vi "SLL DE View Datalog File.vi"(8 "error in(no error)":errorcluster) -> (0 "error Out":errorcluster)   [LabVIEW 2013]
uses:
  Controls/SLL DE Virtual Graph Options.ctl
  Controls/SLL DE Get Plot LV2Global Options.ctl
  Controls/SLL DE Virtual Chart Datalog Driver Options.ctl
  <vilib>/Utility/miscctls.llb/LVAnnotationListTypeDef.ctl
  Controls/SLL DE Get Plot LV2Global Parameters.ctl
panel:
  out "Time :":string="02:30:20 PM"
  out "Date :":string="08-30-2009"
  in  "Import":bool caption="Exit"
  in  "Plot 4":u16(ring) caption="Y-Axis(1)" items=["None"]
  in  "Plot 3":u16(ring) caption="Y-Axis(1)" items=["None"]
  in  "Plot 2":u16(ring) caption="Y-Axis(1)" items=["None"]
  in  "Y-Axis 2":bool=TRUE
  in  "Y-Axis 1":bool=TRUE
  in  "Plot 1":u16(ring) caption="Y-Axis(1)" items=["None"]
  in  "X-Scale":u16(ring) caption="Y-Axis(1)"
  out "Graph":T1(graph)
  in  "Importing File Path":path=path "D:/STI Projects/DAQ Engine/SLL DAQ Engine/Software/Info/Report/Log_08_2009_30_13_15_39.csv"
  in  "Data Cluster":T3={"Record"=FALSE, "Datalog Folder Path"=path "D:/Projects/Projects/Eaton Prop Valve Test Stand/Software/Info/Datalog File Path/Back up.dat", "Graph - Interval b/w Samples"=0, "AI Sampling Rate (Samples/Sec)"=3.0, "Data Log To csv File"=[], "File - Interval b/w Samples"=0, "Time Array"=[], "Graph Mod"=0, "File Mod"=0, "Plot Details"={"Sample Value In"=[], "Plot 1"=FALSE, "Plot 2"=FALSE, "Plot 3"=FALSE, "Plot 4"=FALSE}, "Channel Names"=[]}
  in  "Snap Shot":bool caption="Duplicate SupFile"
  in  "Exit":bool
  in  "Print":bool
  # "Logo"
  # "<Project Name>"
  # "Datalog File Display"
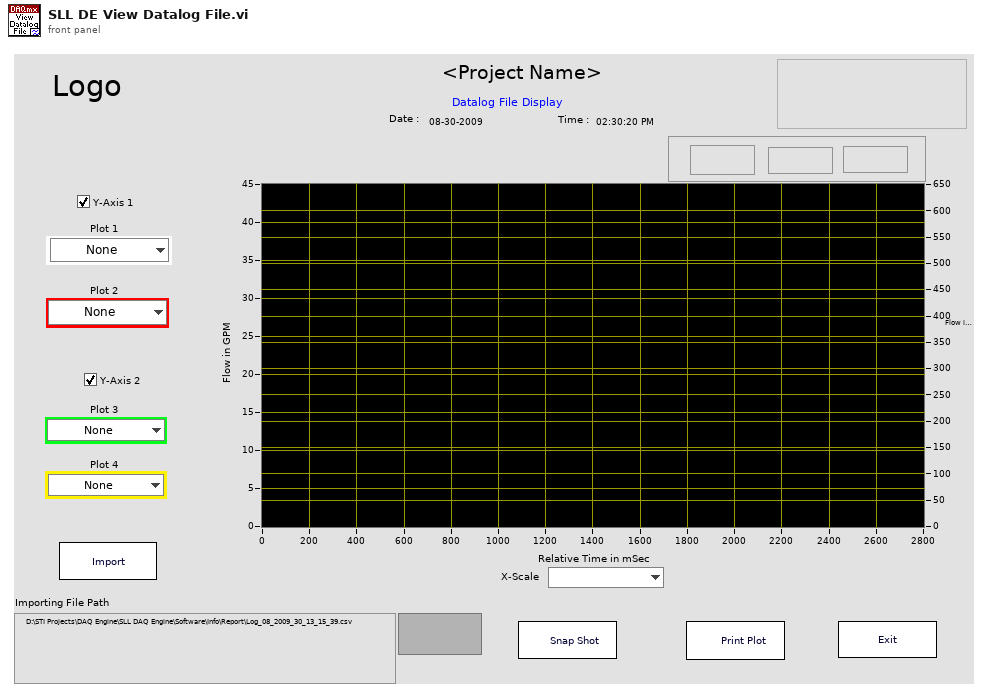
[diagram p1: front panel]
types:
  T1 = cluster{"Sample Value In":sgl[], "Sample Value In":sgl[]}[]
  T2 = typedef "SLL DE Get Plot LV2Global Parameters.ctl" = cluster{"Sample Value In":sgl[][], "Plot 1":bool, "Plot 2":bool, "Plot 3":bool, "Plot 4":bool}
  T3 = cluster{"Record":bool, "Datalog Folder Path":path, "Graph - Interval b/w Samples":i32, "AI Sampling Rate (Samples/Sec)":dbl, "Data Log To csv File":dbl[][], "File - Interval b/w Samples":i32, "Time Array":timestamp[], "Graph Mod":i32, "File Mod":i32, "Plot Details":T2, "Channel Names":string[]}
  T4 = typedef "SLL DE Virtual Graph Options.ctl" = enum16{"Initialize", "Initialize Channel List", "Check Channel Type", "Update Graph Parameters", "Poll Events", "Get Values", "Config Plot", "Plot Ramp", "Datalog", "Add Plot Name", "Enable Record", "Snap Shot", "Restart", "Print Plot", "Error", "Exit"}
  T5 = typedef "SLL DE Get Plot LV2Global Options.ctl" = enum16{"Init", "Get Plot", "Read Plot"}
  T6 = typedef "SLL DE Virtual Chart Datalog Driver Options.ctl" = enum16{"Initialise", "Write Headings", "Write", "Check File Size", "Read", "Clear"}
  T7 = cluster{"Name":string, "Color":u32, "Style":u8, "Point Style":u8, "Name Visible":bool, "Allow Drag":bool, "Annotation Mode":u32, "Plot":i32, "Index":i32, "Position":cluster{"X":dbl, "Y":dbl}, "X Scale":u32, "Y Scale":u32, "Show Arrow":bool, "Lock Name":bool, "Plot Area":i32, "Label Offset":cluster{"X":dbl, "Y":dbl}}[]
  T8 = cluster{"Name":string, "Color":u32, "Style":u8, "Point Style":u8, "Name Visible":bool, "Allow Drag":bool, "Annotation Mode":u32, "Plot":i32, "Index":i32, "Position":cluster{"X":dbl, "Y":dbl}, "X Scale":u32, "Y Scale":u32, "Show Arrow":bool, "Lock Name":bool, "Plot Area":i32, "Label Offset":cluster{"X":dbl, "Y":dbl}}
  T9 = cluster{"Plot 1":string, "Plot 2":string, "Plot 3":string, "Plot 4":string, "X Scale":string, "Y-Axis 2":bool, "Y-Axis 1":bool}
  T10 = typedef "LVAnnotationListTypeDef.ctl" = cluster{"Name":string, "Color":u32, "Style":u8, "Point Style":u8, "Name Visible":bool, "Allow Drag":bool, "Annotation Mode":u32, "Plot":i32, "Index":i32, "Position":cluster{"X":dbl, "Y":dbl}, "X Scale":u32, "Y Scale":u32, "Show Arrow":bool, "Lock Name":bool, "Plot Area":i32, "Label Offset":cluster{"X":dbl, "Y":dbl}}[]
  T11 = typedef "SLL DE List of AI Channel Type.ctl" = enum16{"Pressure", "Flow", "Temperature", "Time Scale", "Voltage", "Current", "Frequency", "Sound", "Speed", "Torque", "Distance", "Channel Type 1", "Channel Type 2", "Channel Type 3"}
  T12 = cluster{"Time Scale":sgl[], "Sample Value In":sgl[]}[]
  T13 = enum16{"Left Button", "Center Button", "Right Button", "Window Close"}
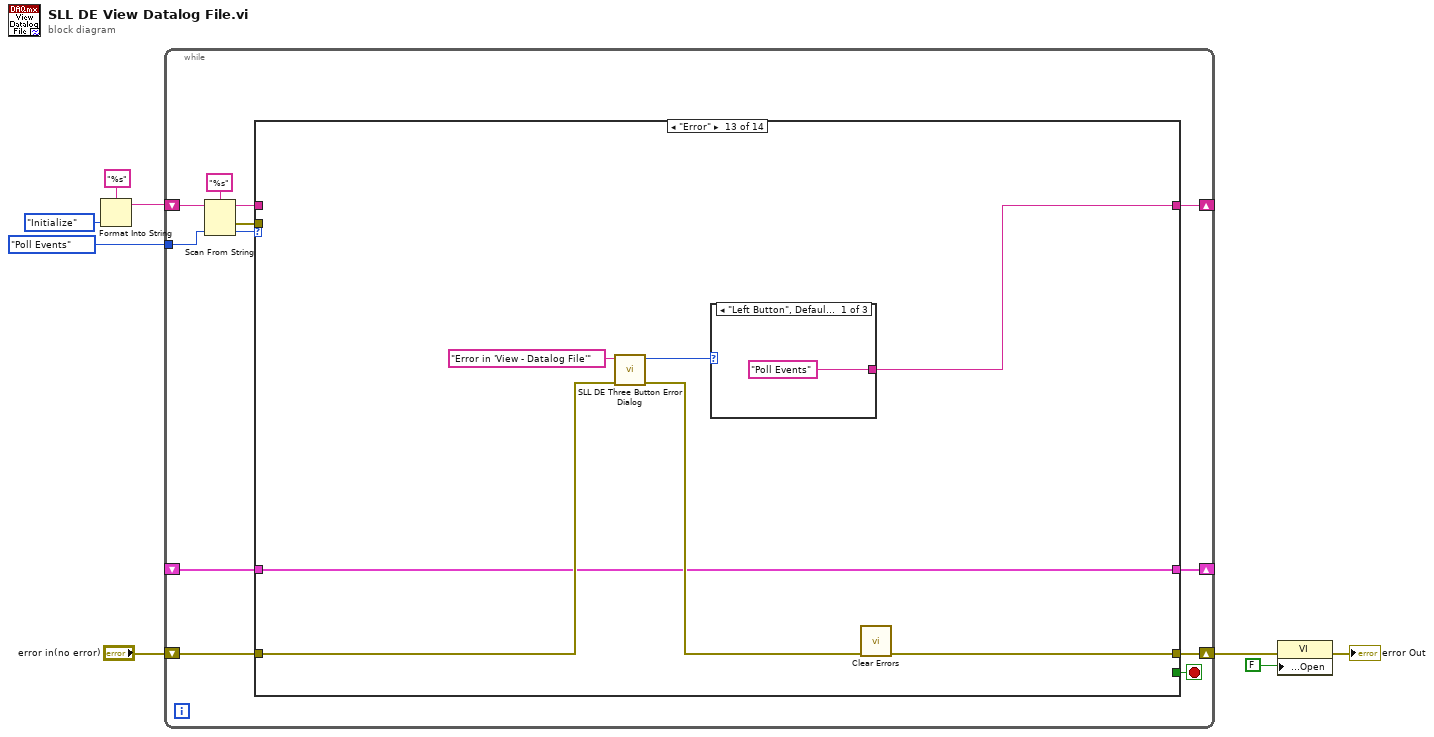
[diagram p0: block diagram]
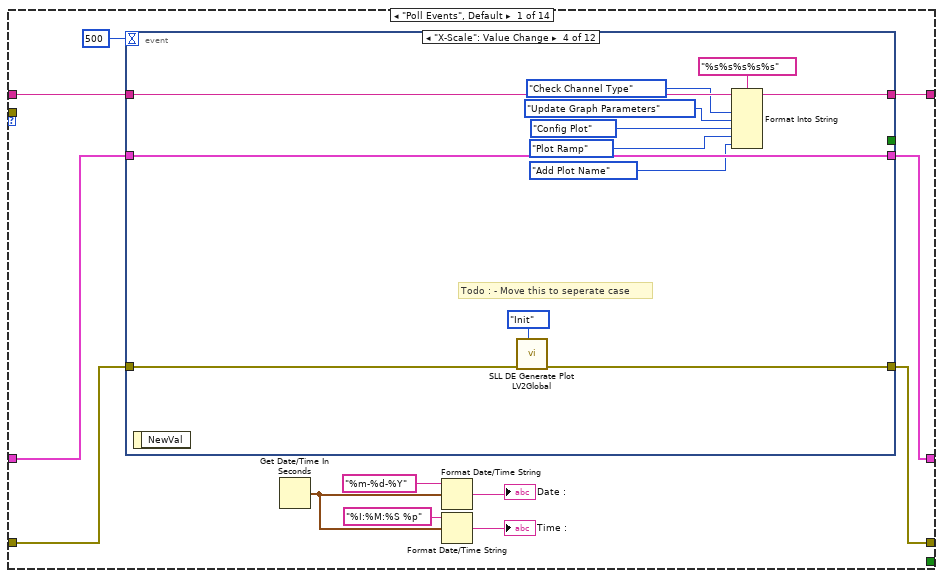
[diagram p2: hidden frame]
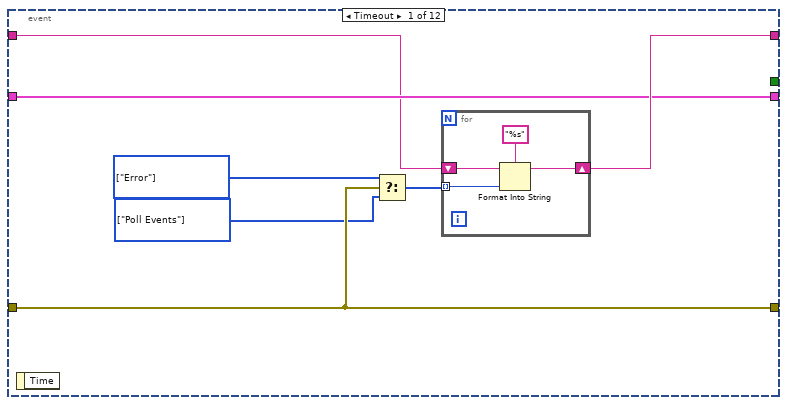
[diagram p3: hidden frame]
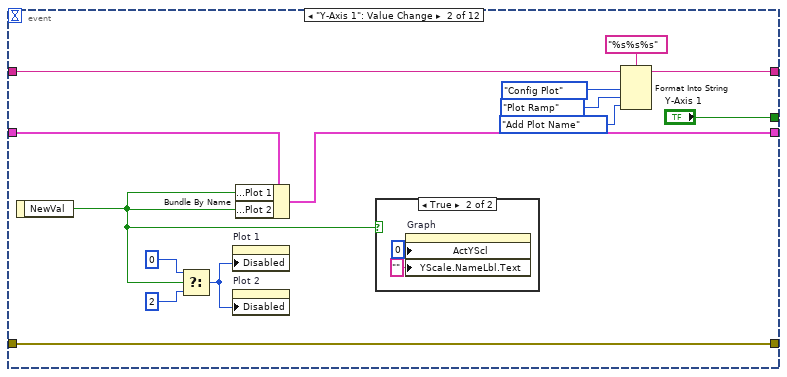
[diagram p4: hidden frame]
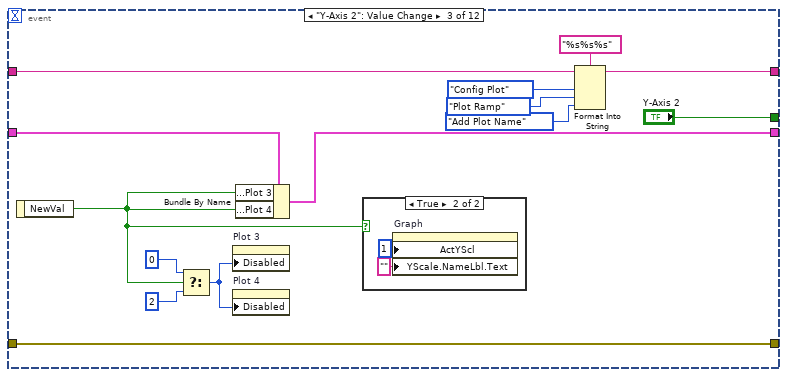
[diagram p6: hidden frame]
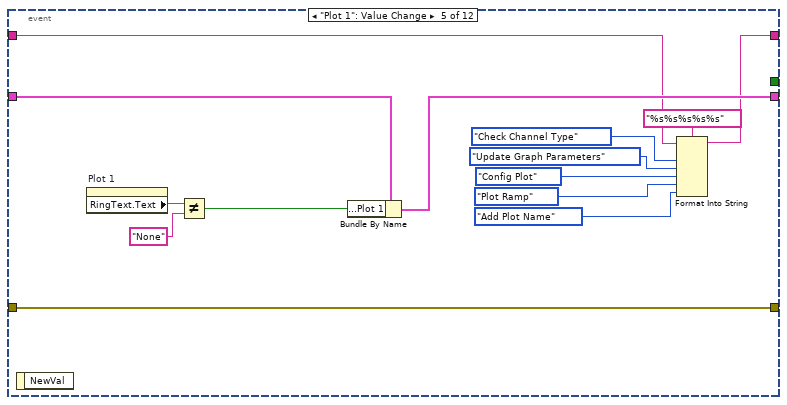
[diagram p8: hidden frame]
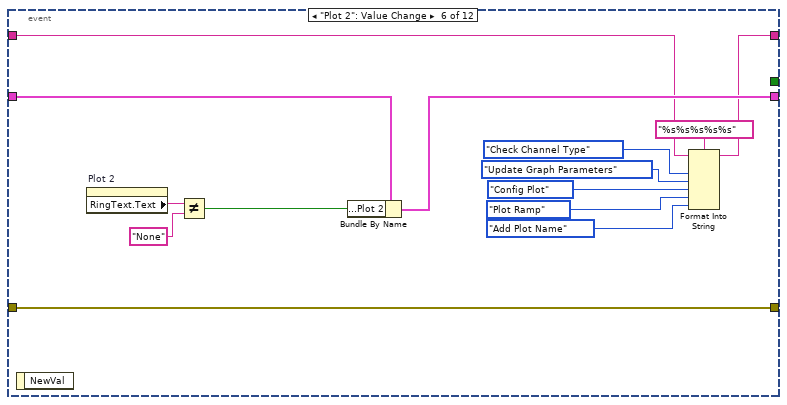
[diagram p9: hidden frame]
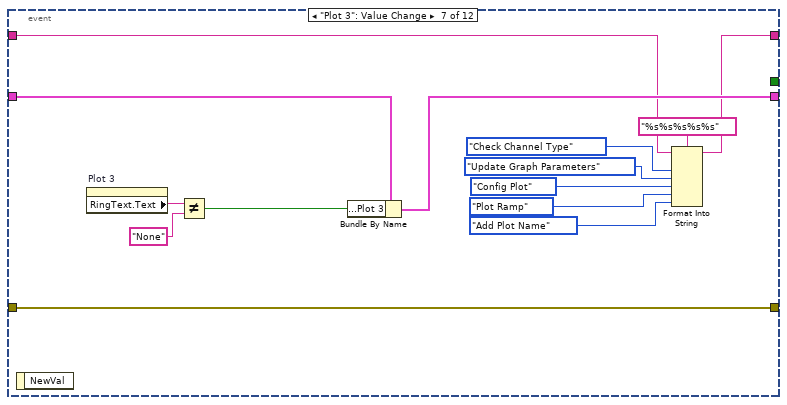
[diagram p10: hidden frame]
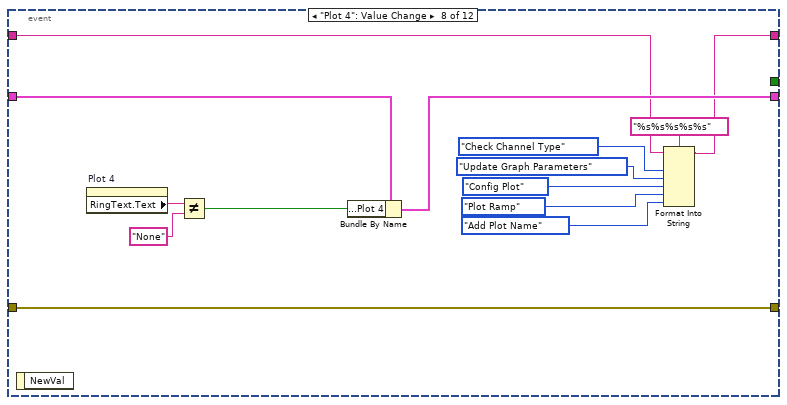
[diagram p11: hidden frame]
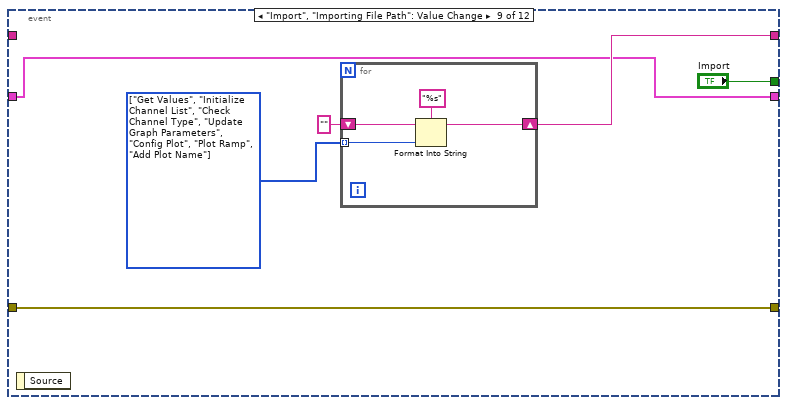
[diagram p12: hidden frame]
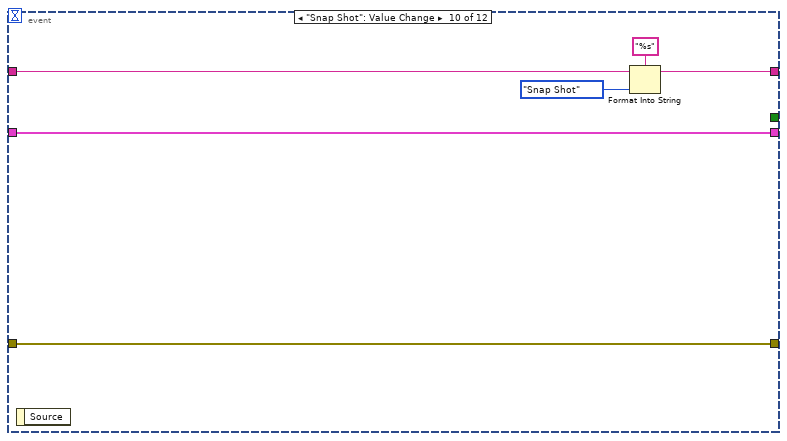
[diagram p13: hidden frame]
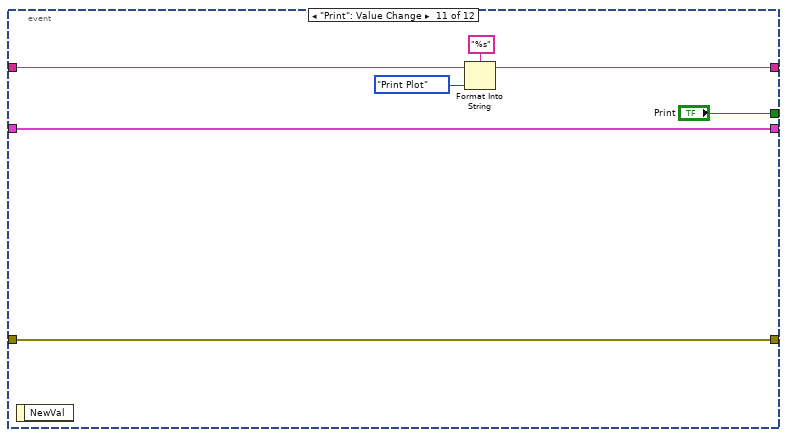
[diagram p14: hidden frame]
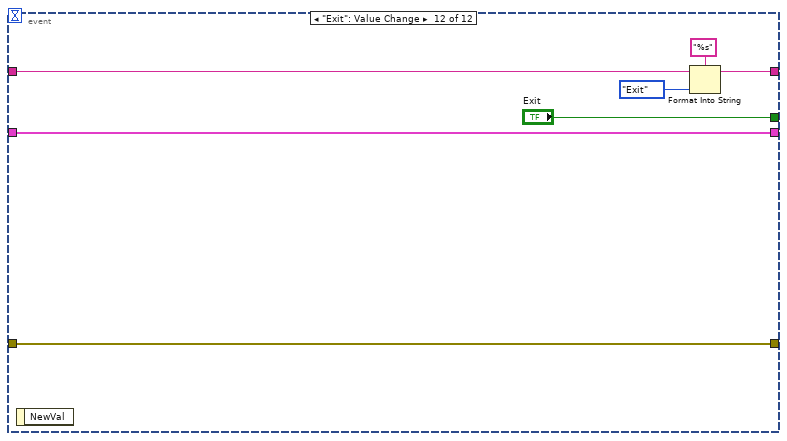
[diagram p15: hidden frame]
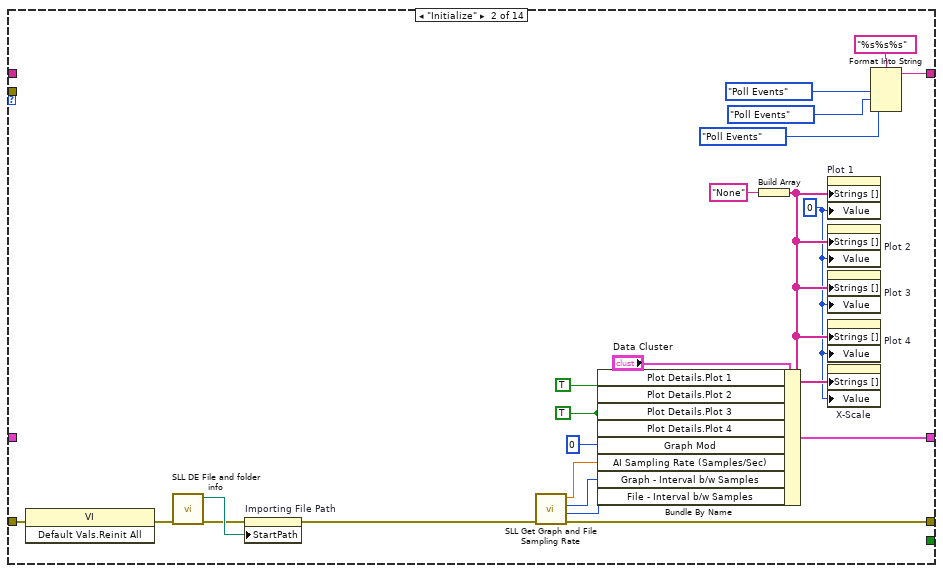
[diagram p16: hidden frame]
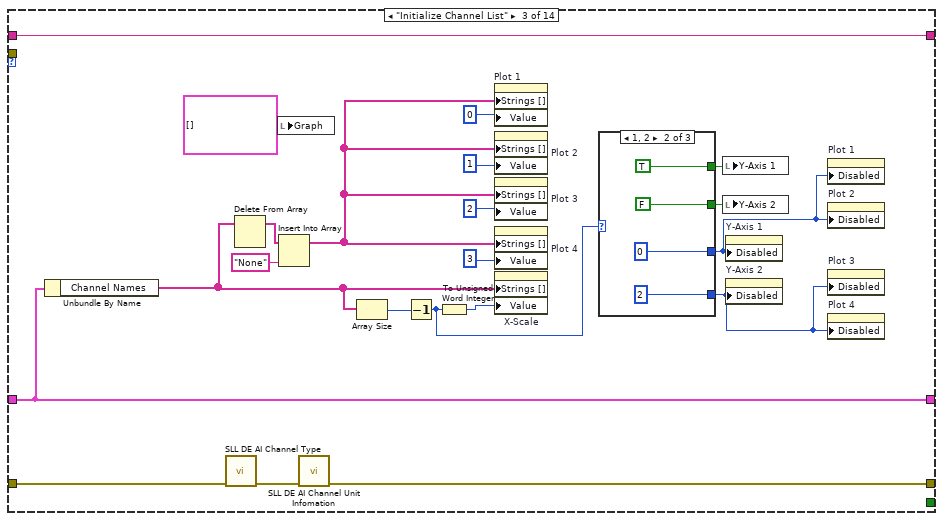
[diagram p17: hidden frame]
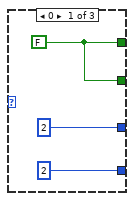
[diagram p18: hidden frame]
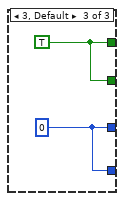
[diagram p19: hidden frame]
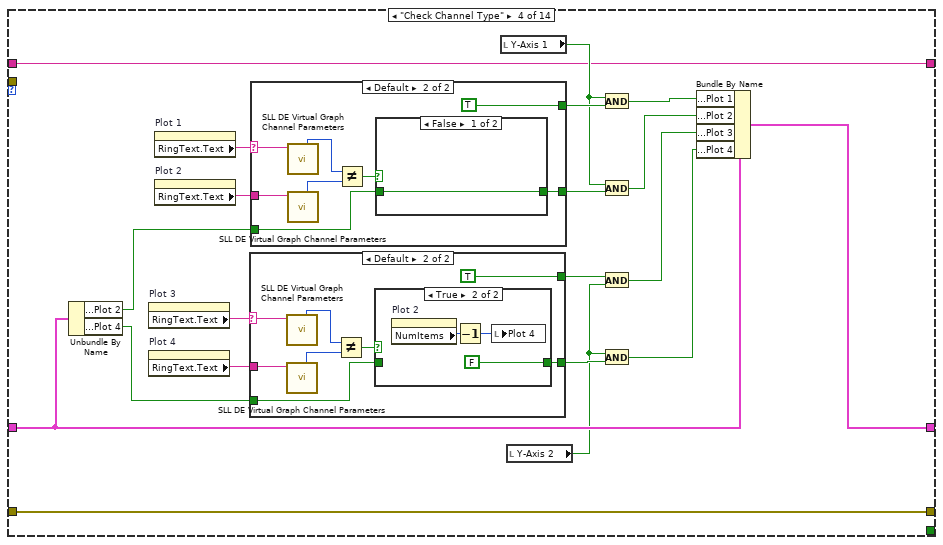
[diagram p20: hidden frame]
diagram:
  n1 = Format Into String(format string="%s", SLL_DE_Virtual_Graph_Options."Initialize" ("SLL DE Virtual Chart Options")) -> (resulting string=w8:string)  [unwired: 2 in, 1 out]
  n2 = while {
    shift-right: [w17] -> _
    shift-left: w8 -> [w20]
    shift-right: [w16] -> _
    shift-left: _ -> [w14]
    shift-right: [w13] -> w6
    shift-left: "error in(no error)" -> [w12]
    tunnel: SLL_DE_Virtual_Graph_Options."Poll Events" ("SLL DE Virtual Chart Options") -> [w10]
    stop <- w15 stop-if-true
    n3 = Scan From String(format string="%s", input string=w20, default 1=w10) -> (remaining string=w18:string, error out=w11:errorcluster, output 1=w19:T4)  [unwired: 2 in, 1 out]
    n4 = case shown="\"Error\"" w19 {
      tunnel: w18 -> [w31 _ w208 w226 w274 w313 w320 w334 w353 w388 w403 w419 _ w437]
      tunnel: [w30 w188 w208 w226 w274 w313 w320 w334 w353 w388 w403 w419 w421 w437] -> w17
      tunnel: [w28 w192 w198 w237 w278 w314 w319 w331 w336 w387 w391 w408 w422 w436] -> w16
      tunnel: [_ _ _ _ _ _ _ _ _ FALSE _ _ _ TRUE] -> w15
      tunnel: w14 -> [w29 _ w198 w238 w278 w312 w319 w331 w336 w387 w391 w408 w422 w436]
      tunnel: [w26 w180 w201 w245 w277 w308 w324 w332 w337 w383 w390 w404 w420 w432] -> w13
      tunnel: w12 -> [w27 w195 w203 w245 w279 w311 w317 w333 w338 w384 w392 w409 w424 w433]
      tunnel: w11 -> [_ _ _ _ _ _ _ _ _ _ _ _ _ _]
      frame "Poll Events", Default {
        n5 = event shown="[3] \"X-Scale\": Value Change" {
          selector: _ -> [_ _ _ _ _ _ _ _ _ _ _ _]
          dyn-events: _ -> [_ _ _ _ _ _ _ _ _ _ _ _]
          timeout: 500 -> [_ _ _ _ _ _ _ _ _ _ _ _]
          tunnel: w31 -> [w34 w52 w62 w80 w90 w104 w117 w130 _ w156 w160 w167]
          tunnel: [w39 w53 w61 w79 w89 w103 w116 w131 w145 w157 w164 w172] -> w30
          tunnel: [_ "Y-Axis 1" "Y-Axis 2" _ _ _ _ _ "Import" _ "Print" "Exit"] -> _
          tunnel: w29 -> [w38 w56 w67 w84 w101 w112 w126 w140 w144 w155 w163 w170]
          tunnel: [w38 w55 w68 w84 w100 w110 w124 w138 w144 w155 w163 w170] -> w28
          tunnel: w27 -> [w37 w50 w69 w86 w99 w111 w125 w139 w149 w154 w162 w169]
          tunnel: [w37 w50 w69 w85 w99 w111 w125 w139 w149 w154 w162 w169] -> w26
          event Timeout {
            w36 = T4[] [enum."Error"] items=["Initialize", "Initialize Channel List", "Check Channel Type", "Update Graph Parameters", "Poll Events", "Get Values", "Config Plot", "Plot Ramp", "Datalog", "Add Plot Name", "Enable Record", "Snap Shot", "Restart", "Print Plot", "Error", "Exit"]
            w35 = T4[] [enum."Poll Events"] items=["Initialize", "Initialize Channel List", "Check Channel Type", "Update Graph Parameters", "Poll Events", "Get Values", "Config Plot", "Plot Ramp", "Datalog", "Add Plot Name", "Enable Record", "Snap Shot", "Restart", "Print Plot", "Error", "Exit"]
            n6 = event-data() -> ()  [unwired: 1 in, 1 out]
            n7 = Select(t=w36, s=w37, f=w35) -> (s? t:f=w33:T4[])
            n8 = for {
              shift-right: [w42] -> w39
              shift-left: w34 -> [w41]
              tunnel: w33 -> [w40] mode=indexing
              n9 = Format Into String(format string="%s", initial string=w41, w40) -> (resulting string=w42:string)  [unwired: 1 in, 1 out]
            }
          }
          event "Y-Axis 1": Value Change {
            n10 = event-data() -> ("NewVal"=w46:bool)  [unwired: 1 in]
            n11 = Select(t=u8 0 ("Disabled"), s=w46, f=u8 2 ("Disabled")) -> (s? t:f=w48:u8)
            n12 = property on="Plot 1" class="Ring (strict)"("Disabled"=w48) -> ()  [unwired: 2 in, 2 out]
            n13 = property on="Plot 2" class="Ring (strict)"("Disabled"=w48) -> ()  [unwired: 2 in, 2 out]
            n14 = Bundle By Name(cluster=w56, "Plot Details.Plot 1"=w46, "Plot Details.Plot 2"=w46) -> (w55:T3)
            n15 = case shown="True" w46 {
              frame False {
              }
              frame True {
                n16 = property on="Graph" class="XYGraph (strict)"("ActYScl"=0 ("Active Y Scale"), "YScale.NameLbl.Text"="" ("Y Scale.Name Label.Text")) -> ()  [unwired: 2 in, 2 out]
              }
            }
            n17 = Format Into String(format string="%s%s%s", initial string=w52, SLL_DE_Virtual_Graph_Options."Config Plot" ("SLL DE Virtual Chart Options"), SLL_DE_Virtual_Graph_Options."Plot Ramp" ("SLL DE Virtual Chart Options"), SLL_DE_Virtual_Graph_Options."Add Plot Name" ("SLL DE Virtual Chart Options")) -> (resulting string=w53:string)  [unwired: 1 in, 1 out]
          }
          event "Y-Axis 2": Value Change {
            n18 = event-data() -> ("NewVal"=w66:bool)  [unwired: 1 in]
            n19 = Select(t=u8 0 ("Disabled"), s=w66, f=u8 2 ("Disabled")) -> (s? t:f=w71:u8)
            n20 = property on="Plot 3" class="Ring (strict)"("Disabled"=w71) -> ()  [unwired: 2 in, 2 out]
            n21 = property on="Plot 4" class="Ring (strict)"("Disabled"=w71) -> ()  [unwired: 2 in, 2 out]
            n22 = Bundle By Name(cluster=w67, "Plot Details.Plot 3"=w66, "Plot Details.Plot 4"=w66) -> (w68:T3)
            n23 = case shown="True" w66 {
              frame False {
              }
              frame True {
                n24 = property on="Graph" class="XYGraph (strict)"("ActYScl"=1 ("Active Y Scale"), "YScale.NameLbl.Text"="" ("Y Scale.Name Label.Text")) -> ()  [unwired: 2 in, 2 out]
              }
            }
            n25 = Format Into String(format string="%s%s%s", initial string=w62, SLL_DE_Virtual_Graph_Options."Config Plot" ("SLL DE Virtual Chart Options"), SLL_DE_Virtual_Graph_Options."Plot Ramp" ("SLL DE Virtual Chart Options"), SLL_DE_Virtual_Graph_Options."Add Plot Name" ("SLL DE Virtual Chart Options")) -> (resulting string=w61:string)  [unwired: 1 in, 1 out]
          }
          event "X-Scale": Value Change {
            # "Todo : - Move this to seperate case"
            n26 = event-data() -> ()  [unwired: 1 in, 1 out]
            n27 = call "SLL DE Generate Plot LV2Global.vi"("Option"=SLL_DE_Get_Plot_LV2Global_Options."Init", "error in (no error)"=w86) -> ("error IO"=w85:errorcluster)  [unwired: 8 in, 1 out]
            n28 = Format Into String(format string="%s%s%s%s%s", initial string=w80, SLL_DE_Virtual_Graph_Options."Check Channel Type" ("SLL DE Virtual Chart Options"), SLL_DE_Virtual_Graph_Options."Update Graph Parameters" ("SLL DE Virtual Chart Options"), SLL_DE_Virtual_Graph_Options."Config Plot" ("SLL DE Virtual Chart Options"), SLL_DE_Virtual_Graph_Options."Plot Ramp" ("SLL DE Virtual Chart Options"), SLL_DE_Virtual_Graph_Options."Add Plot Name" ("SLL DE Virtual Chart Options")) -> (resulting string=w79:string)  [unwired: 1 in, 1 out]
          }
          event "Plot 1": Value Change {
            n29 = event-data() -> ()  [unwired: 1 in, 1 out]
            n30 = property on="Plot 1" class="Ring (strict)"() -> ("RingText.Text"=w98:string)  [unwired: 2 in, 2 out]
            n31 = Not Equal?(x=w98, y="None") -> (x != y?=w96:bool)
            n32 = Bundle By Name(cluster=w101, "Plot Details.Plot 1"=w96) -> (w100:T3)
            n33 = Format Into String(format string="%s%s%s%s%s", initial string=w90, SLL_DE_Virtual_Graph_Options."Check Channel Type" ("SLL DE Virtual Chart Options"), SLL_DE_Virtual_Graph_Options."Update Graph Parameters" ("SLL DE Virtual Chart Options"), SLL_DE_Virtual_Graph_Options."Config Plot" ("SLL DE Virtual Chart Options"), SLL_DE_Virtual_Graph_Options."Plot Ramp" ("SLL DE Virtual Chart Options"), SLL_DE_Virtual_Graph_Options."Add Plot Name" ("SLL DE Virtual Chart Options")) -> (resulting string=w89:string)  [unwired: 1 in, 1 out]
          }
          event "Plot 2": Value Change {
            n34 = event-data() -> ()  [unwired: 1 in, 1 out]
            n35 = property on="Plot 2" class="Ring (strict)"() -> ("RingText.Text"=w115:string)  [unwired: 2 in, 2 out]
            n36 = Not Equal?(x=w115, y="None") -> (x != y?=w113:bool)
            n37 = Bundle By Name(cluster=w112, "Plot Details.Plot 2"=w113) -> (w110:T3)
            n38 = Format Into String(format string="%s%s%s%s%s", initial string=w104, SLL_DE_Virtual_Graph_Options."Check Channel Type" ("SLL DE Virtual Chart Options"), SLL_DE_Virtual_Graph_Options."Update Graph Parameters" ("SLL DE Virtual Chart Options"), SLL_DE_Virtual_Graph_Options."Config Plot" ("SLL DE Virtual Chart Options"), SLL_DE_Virtual_Graph_Options."Plot Ramp" ("SLL DE Virtual Chart Options"), SLL_DE_Virtual_Graph_Options."Add Plot Name" ("SLL DE Virtual Chart Options")) -> (resulting string=w103:string)  [unwired: 1 in, 1 out]
          }
          event "Plot 3": Value Change {
            n39 = event-data() -> ()  [unwired: 1 in, 1 out]
            n40 = property on="Plot 3" class="Ring (strict)"() -> ("RingText.Text"=w129:string)  [unwired: 2 in, 2 out]
            n41 = Not Equal?(x=w129, y="None") -> (x != y?=w127:bool)
            n42 = Bundle By Name(cluster=w126, "Plot Details.Plot 3"=w127) -> (w124:T3)
            n43 = Format Into String(format string="%s%s%s%s%s", initial string=w117, SLL_DE_Virtual_Graph_Options."Check Channel Type" ("SLL DE Virtual Chart Options"), SLL_DE_Virtual_Graph_Options."Update Graph Parameters" ("SLL DE Virtual Chart Options"), SLL_DE_Virtual_Graph_Options."Config Plot" ("SLL DE Virtual Chart Options"), SLL_DE_Virtual_Graph_Options."Plot Ramp" ("SLL DE Virtual Chart Options"), SLL_DE_Virtual_Graph_Options."Add Plot Name" ("SLL DE Virtual Chart Options")) -> (resulting string=w116:string)  [unwired: 1 in, 1 out]
          }
          event "Plot 4": Value Change {
            n44 = event-data() -> ()  [unwired: 1 in, 1 out]
            n45 = property on="Plot 4" class="Ring (strict)"() -> ("RingText.Text"=w143:string)  [unwired: 2 in, 2 out]
            n46 = Not Equal?(x=w143, y="None") -> (x != y?=w141:bool)
            n47 = Bundle By Name(cluster=w140, "Plot Details.Plot 4"=w141) -> (w138:T3)
            n48 = Format Into String(format string="%s%s%s%s%s", initial string=w130, SLL_DE_Virtual_Graph_Options."Check Channel Type" ("SLL DE Virtual Chart Options"), SLL_DE_Virtual_Graph_Options."Update Graph Parameters" ("SLL DE Virtual Chart Options"), SLL_DE_Virtual_Graph_Options."Config Plot" ("SLL DE Virtual Chart Options"), SLL_DE_Virtual_Graph_Options."Plot Ramp" ("SLL DE Virtual Chart Options"), SLL_DE_Virtual_Graph_Options."Add Plot Name" ("SLL DE Virtual Chart Options")) -> (resulting string=w131:string)  [unwired: 1 in, 1 out]
          }
          event "Import", "Importing File Path": Value Change {
            w147 = T4[] [enum."Get Values", enum."Initialize Channel List", enum."Check Channel Type", enum."Update Graph Parameters", enum."Config Plot", enum."Plot Ramp", enum."Add Plot Name"] items=["Initialize", "Initialize Channel List", "Check Channel Type", "Update Graph Parameters", "Poll Events", "Get Values", "Config Plot", "Plot Ramp", "Datalog", "Add Plot Name", "Enable Record", "Snap Shot", "Restart", "Print Plot", "Error", "Exit"]
            n49 = event-data() -> ()  [unwired: 1 in, 1 out]
            n50 = for {
              tunnel: w147 -> [w152] mode=indexing
              shift-right: [w151] -> w145
              shift-left: "" -> [w150]
              n51 = Format Into String(format string="%s", initial string=w150, w152) -> (resulting string=w151:string)  [unwired: 1 in, 1 out]
            }
          }
          event "Snap Shot": Value Change {
            n52 = event-data() -> ()  [unwired: 1 in, 1 out]
            n53 = Format Into String(format string="%s", initial string=w156, SLL_DE_Virtual_Graph_Options."Snap Shot" ("SLL DE Virtual Chart Options")) -> (resulting string=w157:string)  [unwired: 1 in, 1 out]
          }
          event "Print": Value Change {
            n54 = event-data() -> ()  [unwired: 1 in, 1 out]
            n55 = Format Into String(format string="%s", initial string=w160, SLL_DE_Virtual_Graph_Options."Print Plot" ("SLL DE Virtual Chart Options")) -> (resulting string=w164:string)  [unwired: 1 in, 1 out]
          }
          event "Exit": Value Change {
            n56 = event-data() -> ()  [unwired: 1 in, 1 out]
            n57 = Format Into String(format string="%s", initial string=w167, SLL_DE_Virtual_Graph_Options."Exit" ("SLL DE Virtual Chart Options")) -> (resulting string=w172:string)  [unwired: 1 in, 1 out]
          }
        }
        n58 = Get Date/Time In Seconds() -> (seconds since 1Jan1904=w23:timestamp)
        n59 = Format Date/Time String(time format string (%c)="%m-%d-%Y", seconds (now)=w23) -> (date/time string=→"Date :":string)  [unwired: 1 in]
        n60 = Format Date/Time String(time format string (%c)="%I:%M:%S %p", seconds (now)=w23) -> (date/time string=→"Time :":string)  [unwired: 1 in]
      }
      frame "Initialize" {
        w174 = 0
        w185 = TRUE ("Data Cluster 2.Plot 1")
        n61 = invoke class="VI" method="Default Vals.Reinit All"(error in=w195) -> (error out=w194:errorcluster)  [unwired: 2 in, 2 out]
        n62 = call "SLL DE File and folder info.vi"("error in (no error)"=w194) -> ("error out"=w178:errorcluster, "Report path"=w179:path)  [unwired: 5 in, 4 out]
        n63 = property on="Importing File Path" class="Path"(error in=w178, "StartPath"=w179) -> (error out=w177:errorcluster)  [unwired: 1 in, 1 out]
        n64 = call "SLL Get Graph and File Sampling Rate.vi"("error in (no error)"=w177) -> ("error out"=w180:errorcluster, "File - Interval b/w Samples"=w182:i32, "Graph - Interval b/w Samples"=w183:i32, "AI Sampling Rate (Samples/Sec)"=w184:dbl)  [unwired: 7 in]
        n65 = Bundle By Name(cluster="Data Cluster", "Plot Details.Plot 1"=TRUE ("Data Cluster 2.Plot 1"), "Plot Details.Plot 2"=w185, "Plot Details.Plot 3"=w185, "Plot Details.Plot 4"=w185, "Graph Mod"=0 ("Mod"), "AI Sampling Rate (Samples/Sec)"=w184, "Graph - Interval b/w Samples"=w183, "File - Interval b/w Samples"=w182) -> (w192:T3)
        n66 = Build Array("None") -> (w175:string[])
        n67 = property on="Plot 1" class="Ring (strict)"("Strings []"=w175, "Value"=w174) -> ()  [unwired: 2 in, 2 out]
        n68 = property on="Plot 2" class="Ring (strict)"("Strings []"=w175, "Value"=w174) -> ()  [unwired: 2 in, 2 out]
        n69 = property on="Plot 3" class="Ring (strict)"("Strings []"=w175, "Value"=w174) -> ()  [unwired: 2 in, 2 out]
        n70 = property on="Plot 4" class="Ring (strict)"("Strings []"=w175, "Value"=w174) -> ()  [unwired: 2 in, 2 out]
        n71 = property on="X-Scale" class="Ring (strict)"("Strings []"=w175, "Value"=w174) -> ()  [unwired: 2 in, 2 out]
        n72 = Format Into String(format string="%s%s%s", SLL_DE_Virtual_Graph_Options."Poll Events" ("SLL DE Virtual Chart Options"), SLL_DE_Virtual_Graph_Options."Poll Events" ("SLL DE Virtual Chart Options"), SLL_DE_Virtual_Graph_Options."Poll Events" ("SLL DE Virtual Chart Options")) -> (resulting string=w188:string)  [unwired: 2 in, 1 out]
      }
      frame "Initialize Channel List" {
        n73 = Unbundle By Name(w198) -> ("Channel Names"=w197:string[])
        n74 = call "SLL DE AI Channel Type.vi"("error in (no error)"=w203) -> ("error out"=w202:errorcluster)  [unwired: 7 in, 3 out]
        n75 = Delete From Array(array=w197) -> (array with subset deleted=w196:string[])  [unwired: 2 in, 1 out]
        n76 = local write "Graph"(T1 [] ("Graph")) -> ()
        n77 = Insert Into Array(array=w196, new element="None") -> (w210:string[])  [unwired: 1 in]
        n78 = call "SLL DE AI Channel Unit Infomation.vi"("error in (no error)"=w202) -> ("error out"=w201:errorcluster)  [unwired: 9 in, 1 out]
        n79 = Array Size(array=w197) -> (size(s)=w211:i32)
        n80 = Decrement(x=w211) -> (x-1=w213:i32)
        n81 = To Unsigned Word Integer(number=w213) -> (unsigned 16bit integer=w212:u16)
        n82 = property on="Plot 1" class="Ring (strict)"("Strings []"=w210, "Value"=u16 0) -> ()  [unwired: 2 in, 2 out]
        n83 = property on="Plot 2" class="Ring (strict)"("Strings []"=w210, "Value"=u16 1) -> ()  [unwired: 2 in, 2 out]
        n84 = property on="Plot 3" class="Ring (strict)"("Strings []"=w210, "Value"=u16 2) -> ()  [unwired: 2 in, 2 out]
        n85 = property on="Plot 4" class="Ring (strict)"("Strings []"=w210, "Value"=u16 3) -> ()  [unwired: 2 in, 2 out]
        n86 = property on="X-Scale" class="Ring (strict)"("Strings []"=w197, "Value"=w212) -> ()  [unwired: 2 in, 2 out]
        n87 = case shown="1, 2" w213 {
          tunnel: [w219 TRUE w225] -> w214
          tunnel: [w219 FALSE w225] -> w215
          tunnel: [u8 2 ("Disabled") u8 0 ("Disabled") w224] -> w200
          tunnel: [u8 2 ("Disabled") u8 2 ("Disabled") w224] -> w199
          frame 0 {
            w219 = FALSE
          }
          frame 1, 2 {
          }
          frame 3, Default {
            w224 = u8 0 ("Disabled")
            w225 = TRUE
          }
        }
        n88 = local write "Y-Axis 1"(w214) -> ()
        n89 = local write "Y-Axis 2"(w215) -> ()
        n90 = property on="Y-Axis 1" class="Bool (strict)"("Disabled"=w200) -> ()  [unwired: 2 in, 2 out]
        n91 = property on="Y-Axis 2" class="Bool (strict)"("Disabled"=w199) -> ()  [unwired: 2 in, 2 out]
        n92 = property on="Plot 1" class="Ring (strict)"("Disabled"=w200) -> ()  [unwired: 2 in, 2 out]
        n93 = property on="Plot 2" class="Ring (strict)"("Disabled"=w200) -> ()  [unwired: 2 in, 2 out]
        n94 = property on="Plot 3" class="Ring (strict)"("Disabled"=w199) -> ()  [unwired: 2 in, 2 out]
        n95 = property on="Plot 4" class="Ring (strict)"("Disabled"=w199) -> ()  [unwired: 2 in, 2 out]
      }
      frame "Check Channel Type" {
        n96 = Unbundle By Name(w238) -> ("Plot Details.Plot 2"=w240:bool, "Plot Details.Plot 4"=w239:bool)
        n97 = property on="Plot 3" class="Ring (strict)"() -> ("RingText.Text"=w242:string)  [unwired: 2 in, 2 out]
        n98 = property on="Plot 4" class="Ring (strict)"() -> ("RingText.Text"=w241:string)  [unwired: 2 in, 2 out]
        n99 = property on="Plot 1" class="Ring (strict)"() -> ("RingText.Text"=w243:string)  [unwired: 2 in, 2 out]
        n100 = property on="Plot 2" class="Ring (strict)"() -> ("RingText.Text"=w244:string)  [unwired: 2 in, 2 out]
        n101 = case shown="Default" w242 {
          selector: w242 -> [_ w251]
          tunnel: w241 -> [_ w255]
          tunnel: [FALSE TRUE] -> w230
          tunnel: [w246 w249] -> w229
          tunnel: w239 -> [w246 w248]
          frame "None" {
          }
          frame Default {
            n102 = call "SLL DE Virtual Graph Channel Parameters.vi"("Virtual Channel Name"=w251) -> ("Channel Type"=w254:T11)  [unwired: 5 in, 5 out]
            n103 = call "SLL DE Virtual Graph Channel Parameters.vi"("Virtual Channel Name"=w255) -> ("Channel Type"=w253:T11)  [unwired: 5 in, 5 out]
            n104 = Not Equal?(x=w254, y=w253) -> (x != y?=w252:bool)
            n105 = case shown="True" w252 {
              tunnel: [w256 FALSE] -> w249
              tunnel: w248 -> [w256 _]
              frame False {
              }
              frame True {
                n106 = property on="Plot 2" class="Ring (strict)"() -> ("NumItems"=w258:u32)  [unwired: 2 in, 2 out]
                n107 = Decrement(x=w258) -> (x-1=w257:u32)
                n108 = local write "Plot 4"(w257) -> ()
              }
            }
          }
        }
        n109 = case shown="Default" w243 {
          selector: w243 -> [_ w265]
          tunnel: w244 -> [_ w269]
          tunnel: [FALSE TRUE] -> w235
          tunnel: [w260 w263] -> w234
          tunnel: w240 -> [w260 w262]
          frame "None" {
          }
          frame Default {
            n110 = call "SLL DE Virtual Graph Channel Parameters.vi"("Virtual Channel Name"=w265) -> ("Channel Type"=w268:T11)  [unwired: 5 in, 5 out]
            n111 = call "SLL DE Virtual Graph Channel Parameters.vi"("Virtual Channel Name"=w269) -> ("Channel Type"=w267:T11)  [unwired: 5 in, 5 out]
            n112 = Not Equal?(x=w268, y=w267) -> (x != y?=w266:bool)
            n113 = case shown="False" w266 {
              tunnel: [w270 FALSE] -> w263
              tunnel: w262 -> [w270 _]
              frame False {
              }
              frame True {
                n114 = property on="Plot 2" class="Ring (strict)"() -> ("NumItems"=w272:u32)  [unwired: 2 in, 2 out]
                n115 = Decrement(x=w272) -> (x-1=w271:u32)
                n116 = local write "Plot 2"(w271) -> ()
              }
            }
          }
        }
        n117 = local read "Y-Axis 1"() -> (w233:bool)
        n118 = local read "Y-Axis 2"() -> (w228:bool)
        n119 = And(x=w233, y=w235) -> (x .and. y?=w236:bool)
        n120 = And(x=w233, y=w234) -> (x .and. y?=w232:bool)
        n121 = And(x=w230, y=w228) -> (x .and. y?=w231:bool)
        n122 = And(x=w228, y=w229) -> (x .and. y?=w227:bool)
        n123 = Bundle By Name(cluster=w238, "Plot Details.Plot 1"=w236, "Plot Details.Plot 2"=w232, "Plot Details.Plot 3"=w231, "Plot Details.Plot 4"=w227) -> (w237:T3)
      }
      frame "Update Graph Parameters" {
        n124 = property on="X-Scale" class="Ring (strict)"(error in=w279) -> (error out=w276:errorcluster, "RingText.Text"=w275:string)  [unwired: 1 in, 1 out]
        n125 = property on="Plot 1" class="Ring (strict)"(error in=w279) -> (error out=w280:errorcluster, "RingText.Text"=w281:string)  [unwired: 1 in, 1 out]
        n126 = property on="Plot 3" class="Ring (strict)"(error in=w279) -> ("RingText.Text"=w282:string)  [unwired: 1 in, 2 out]
        n127 = Build Array(w281, w282) -> (w283:string[])
        n128 = case shown="Default" w275 {
          selector: w275 -> [_ w286]
          tunnel: w276 -> [w285 w288]
          frame "Time Scale" {
            n129 = property on="Graph" class="XYGraph (strict)"(error in=w285, "XScale.NameLbl.Text"="Relative Time in mSec" ("X Scale.Name Label.Text")) -> ()  [unwired: 1 in, 2 out]
          }
          frame Default {
            n130 = call "SLL DE Virtual Graph Channel Parameters.vi"("error in (no error)"=w288, "Virtual Channel Name"=w286) -> ("error out"=w287:errorcluster, "Maximum Value"=w290:dbl, "Minimum Value"=w291:dbl, "Graph Name Label"=w292:string, "Increment"=w289:dbl)  [unwired: 4 in, 1 out]
            n131 = property on="Graph" class="XYGraph (strict)"(error in=w287, "XScale.NameLbl.Text"=w292, "XScale.Minimum"=w291, "XScale.Maximum"=w290, "XScale.Increment"=w289) -> ()  [unwired: 1 in, 2 out]
          }
        }
        n132 = for {
          tunnel: w283 -> [w297] mode=indexing
          shift-right: [w296] -> w277
          shift-left: w280 -> [w295]
          i -> [w298]
          n133 = property on="Graph" class="XYGraph (strict)"(error in=w295, "ActYScl"=w298) -> (error out=w294:errorcluster)  [unwired: 1 in, 1 out]
          n134 = call "SLL DE Virtual Graph Channel Parameters.vi"("error in (no error)"=w294, "Virtual Channel Name"=w297) -> ("error out"=w293:errorcluster, "Graph Name Label"=w299:string)  [unwired: 4 in, 4 out]
          n135 = property on="Graph" class="XYGraph (strict)"(error in=w293, "YScale.NameLbl.Text"=w299) -> (error out=w296:errorcluster)  [unwired: 1 in, 1 out]
        }
      }
      frame "Get Values" {
        n136 = call "SLL DE csv File Driver.vi"("Datalog Driver Cases"=SLL_DE_Virtual_Chart_Datalog_Driver_Options."Initialise", "error in(no error)"=w311, "Datalog path (use dialog)"="Importing File Path") -> ("error out"=w310:errorcluster)  [unwired: 4 in, 4 out]
        n137 = call "SLL DE csv File Driver.vi"("Datalog Driver Cases"=SLL_DE_Virtual_Chart_Datalog_Driver_Options."Read", "error in(no error)"=w310) -> ("error out"=w309:errorcluster, "Data Out"=w304:dbl[][], "Channel Names"=w302:string[])  [unwired: 5 in, 2 out]
        n138 = call "SLL DE csv File Driver.vi"("Datalog Driver Cases"=SLL_DE_Virtual_Chart_Datalog_Driver_Options."Clear", "error in(no error)"=w309) -> ("error out"=w308:errorcluster)  [unwired: 5 in, 4 out]
        n139 = To Single Precision Float(number=w304) -> (single precision float=w303:sgl[][])
        n140 = Transpose 2D Array(2D array=w303) -> (transposed array=w300:sgl[][])
        n141 = Bundle By Name(cluster=w312, "Plot Details.Sample Value In"=w300, "Channel Names"=w302) -> (w314:T3)
      }
      frame "Config Plot" {
        n142 = call "SLL DE Generate Plot LV2Global.vi"("Option"=SLL_DE_Get_Plot_LV2Global_Options."Init", "error in (no error)"=w317) -> ("error IO"=w316:errorcluster)  [unwired: 8 in, 1 out]
        n143 = control-ref of="X-Scale"() -> (w315:refnum<vi>)
        n144 = Unbundle By Name(w319) -> ("Plot Details"=w322:T2)
        n145 = Build Array("Plot 1", "Plot 2", "Plot 3", "Plot 4") -> (w323:u16[])
        n146 = call "SLL DE Generate Plot LV2Global.vi"("Option"=SLL_DE_Get_Plot_LV2Global_Options."Get Plot", "error in (no error)"=w316, "X-Scale"=w315, "Plots"=w323, "Data Cluster"=w322) -> ("error IO"=w324:errorcluster)  [unwired: 5 in, 1 out]
      }
      frame "Plot Ramp" {
        # "Based on the configure plot details in both the axis, the \nramp detail for the particular channels corresponding to \nthe axis details will be plotted."
        n147 = call "SLL DE Generate Plot LV2Global.vi"("Option"=SLL_DE_Get_Plot_LV2Global_Options."Read Plot", "error in (no error)"=w333) -> ("error IO"=w332:errorcluster, "Plot data array"=→"Graph":T12)  [unwired: 8 in]
      }
      frame "Add Plot Name" {
        n148 = property on="Plot 1" class="Ring (strict)"() -> ("RingText.Text"=w347:string)  [unwired: 2 in, 2 out]
        n149 = property on="Plot 2" class="Ring (strict)"() -> ("RingText.Text"=w348:string)  [unwired: 2 in, 2 out]
        n150 = property on="Plot 3" class="Ring (strict)"() -> ("RingText.Text"=w349:string)  [unwired: 2 in, 2 out]
        n151 = property on="Plot 4" class="Ring (strict)"() -> ("RingText.Text"=w350:string)  [unwired: 2 in, 2 out]
        n152 = call "SLL DE Generate Plot LV2Global.vi"("Option"=SLL_DE_Get_Plot_LV2Global_Options."Read Plot", "error in (no error)"=w338) -> ("error IO"=w337:errorcluster, "Plot data array"=w345:T12)  [unwired: 8 in]
        n153 = Unbundle By Name(w336) -> ("Plot Details.Plot 1"=w340:bool, "Plot Details.Plot 2"=w341:bool, "Plot Details.Plot 3"=w342:bool, "Plot Details.Plot 4"=w343:bool)
        n154 = Build Array(w340, w341, w342, w343) -> (w344:bool[])
        n155 = Build Array(w347, w348, w349, w350) -> (w351:string[])
        n156 = for {
          tunnel: w344 -> [w359] mode=indexing
          tunnel: w345 -> [w360] mode=indexing
          shift-right: [w357] -> w335
          shift-left: T7 [] -> [w354]
          tunnel: u32[] [16777215, 16728642, 982784, 16776704] ("Array") -> [w356] mode=indexing
          tunnel: w351 -> [w355] mode=indexing
          i -> [w358]
          n157 = case shown="True" w359 {
            tunnel: w360 -> [_ w377]
            tunnel: w358 -> [_ w362]
            tunnel: [w361 w372] -> w357
            tunnel: w356 -> [_ w380]
            tunnel: w355 -> [_ w379]
            tunnel: w354 -> [w361 w378]
            frame False {
            }
            frame True {
              n158 = Unbundle(w377) -> ("Time Scale"=w365:sgl[], "Sample Value In"=w374:sgl[])
              n159 = Less Or Equal?(x=w362, y=1) -> (x <= y?=w370:bool)
              n160 = Array Size(array=w365) -> (size(s)=w364:i32)
              n161 = Quotient & Remainder(x=w364, y=2) -> (floor(x/y)=w373:i32)  [unwired: 1 out]
              n162 = Select(t=0, s=w370, f=1) -> (s? t:f=w367:i32)
              n163 = Index Array(array=w365, index=w373) -> (element=w376:sgl)
              n164 = Index Array(array=w374, index=w373) -> (element=w375:sgl)
              n165 = Bundle By Name(cluster=T8 {"Name"="", "Color"=0, "Style"=4, "Point Style"=0, "Name Visible"=TRUE, "Allow Drag"=TRUE, "Annotation Mode"=0, "Plot"=0, "Index"=0, "Position"={"X"=0.0, "Y"=0.0}, "X Scale"=0, "Y Scale"=0, "Show Arrow"=TRUE, "Lock Name"=FALSE, "Plot Area"=0, "Label Offset"={"X"=0.0, "Y"=0.0}} ("element"), "Name"=w379, "Color"=w380, "Position.X"=w376, "Position.Y"=w375, "Y Scale"=w367, "Plot"=w362) -> (w381:T8)
              n166 = Build Array (concatenate)(w378, w381) -> (w372:T7)
            }
          }
        }
        n167 = property on="Graph" class="XYGraph (strict)"("AnntList"=w335) -> ()  [unwired: 2 in, 2 out]
      }
      frame "Restart" {
        n168 = call "SLL DE Generate Plot LV2Global.vi"("Option"=SLL_DE_Get_Plot_LV2Global_Options."Init", "error in (no error)"=w384) -> ("error IO"=w383:errorcluster)  [unwired: 8 in, 1 out]
        n169 = Request Deallocation(TRUE ("flag")) -> ()
        n170 = local write "Graph"(T1 [] ("Graph")) -> ()
      }
      frame "Snap Shot" {
        n171 = call "SLL DE File and folder info.vi"("error in (no error)"=w392) -> ("error out"=w390:errorcluster, "Report path"=w394:path)  [unwired: 5 in, 4 out]
        n172 = Get Date/Time In Seconds() -> (seconds since 1Jan1904=w396:timestamp)
        n173 = Format Date/Time String(time format string (%c)="%m_%Y_%d_%H_%M_%S", seconds (now)=w396) -> (date/time string=w400:string)  [unwired: 1 in]
        n174 = Concatenate Strings("Log_" ("string"), w400, ".bmp" ("string")) -> (w395:string)
        n175 = Build Path(base path=w394, name or relative path=w395) -> (appended path=w393:path)
        n176 = invoke on="Graph" class="XYGraph (strict)" method="Export Image Color"("File Type"=enum32{"BMP", "EPS", "EMF", "PICT"}."BMP", "Target"=enum32{"File", "Clipboard"}."File", "Path"=w393) -> ()  [unwired: 5 in, 8 out]
      }
      frame "Print Plot" {
        n177 = property on="Plot 1" class="Ring (strict)"() -> ("RingText.Text"=w417:string)  [unwired: 2 in, 2 out]
        n178 = property on="Plot 2" class="Ring (strict)"() -> ("RingText.Text"=w416:string)  [unwired: 2 in, 2 out]
        n179 = property on="Plot 3" class="Ring (strict)"() -> ("RingText.Text"=w415:string)  [unwired: 2 in, 2 out]
        n180 = property on="Plot 4" class="Ring (strict)"() -> ("RingText.Text"=w414:string)  [unwired: 2 in, 2 out]
        n181 = property on="X-Scale" class="Ring (strict)"() -> ("RingText.Text"=w413:string)  [unwired: 2 in, 2 out]
        n182 = local read "Y-Axis 2"() -> (w411:bool)
        n183 = local read "Y-Axis 1"() -> (w412:bool)
        n184 = Bundle By Name(cluster=T9 {"Plot 1"="", "Plot 2"="", "Plot 3"="", "Plot 4"="", "X Scale"="", "Y-Axis 2"=FALSE, "Y-Axis 1"=FALSE} ("Parameters"), "Plot 1"=w417, "Plot 2"=w416, "Plot 3"=w415, "Plot 4"=w414, "X Scale"=w413, "Y-Axis 2"=w411, "Y-Axis 1"=w412) -> (w407:T9)
        n185 = call "SLL DE Generate Plot LV2Global.vi"("Option"=SLL_DE_Get_Plot_LV2Global_Options."Read Plot", "error in (no error)"=w409) -> ("error IO"=w405:errorcluster, "Plot data array"=w406:T12)  [unwired: 8 in]
        n186 = call "SLL DE Print Chart.vi"("error in (no error)"=w405, "Plot data array"=w406, "Parameters"=w407) -> ("error out"=w404:errorcluster)  [unwired: 8 in]
      }
      frame "Error" {
        n187 = call "SLL DE Three Button Error Dialog.vi"("Error In"=w424, "Window Title"="Error in 'View - Datalog File'") -> ("Error Out"=w423:errorcluster, "Which Button?"=w426:T13)  [unwired: 8 in]
        n188 = case shown="\"Left Button\", Default" w426 {
          tunnel: ["Poll Events" ("Window Title") "Initialize" ("Window Title") "Exit" ("Window Title")] -> w421
          frame "Left Button", Default {
          }
          frame "Center Button" {
          }
          frame "Right Button" {
          }
        }
        n189 = call <vilib>:"Clear Errors.vi"("error in (no error)"=w423) -> ("error out"=w420:errorcluster)  [unwired: 5 in, 1 out]
      }
      frame "Exit" {
        n190 = property on="Graph" class="XYGraph (strict)"("AnntList"=T10 [] ("Annotation List")) -> ()  [unwired: 2 in, 2 out]
        n191 = call "SLL DE Generate Plot LV2Global.vi"("Option"=SLL_DE_Get_Plot_LV2Global_Options."Init", "error in (no error)"=w433) -> ("error IO"=w432:errorcluster)  [unwired: 8 in, 1 out]
        n192 = Request Deallocation(TRUE ("flag")) -> ()
        n193 = local write "Graph"(T1 [] ("Graph")) -> ()
      }
    }
  }
  n194 = property class="VI"(error in=w6, "Front Panel.Open"=FALSE ("Front Panel Window:Open")) -> (error out=→"error Out":errorcluster)  [unwired: 1 in, 1 out]
